vi "Async VI Control_Stop Processes.vi"(5 "Iterations":i32=39, 11 "VI Refs":refnum<vi>[](array[refnum])) -> ()   [LabVIEW 2021, in "CANOpen Addon Engine.lvlib"]
uses:
  CANOpen Addon Engine.lvlib
panel:
  out "error out":errorcluster
  out "States":T1(array[ring])
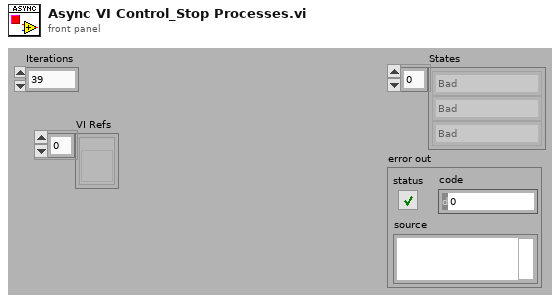
[diagram p1: front panel]
types:
  T1 = enum32{"Bad", "Idle", "Run top level", "Running"}[]
  T2 = enum32{"Bad", "Idle", "Run top level", "Running"}
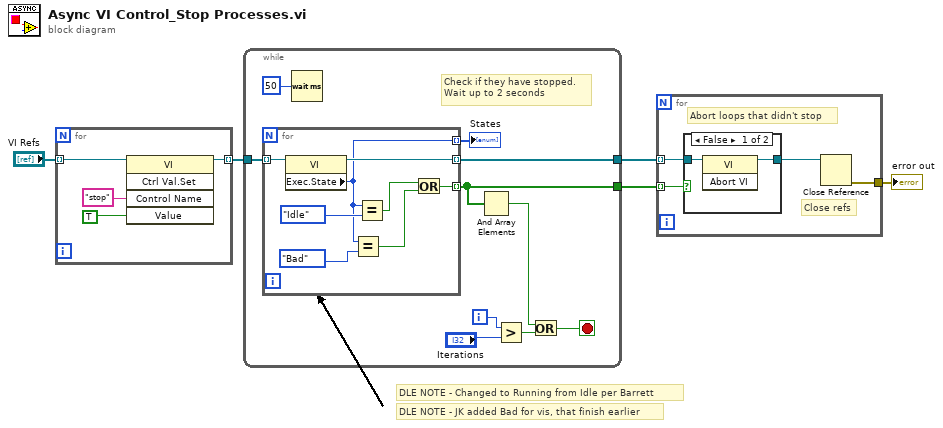
[diagram p0: block diagram]
diagram:
  # "DLE NOTE - JK added Bad for vis, that finish earlier"
  # "DLE NOTE - Changed to Running from Idle per Barrett"
  n1 = for {
    tunnel: "VI Refs" -> [w9] mode=indexing
    tunnel: [w7] -> w4 mode=indexing
    n2 = invoke class="VI" method="Ctrl Val.Set"(reference=w9, "Control Name"="stop", "Value"=TRUE ("force destroy? (F)")) -> (reference out=w7:refnum<vi>)  [unwired: 2 in, 4 out]
  }
  n3 = while {
    tunnel: w4 -> [w18]
    tunnel: [w17] -> w2
    tunnel: [w12] -> w3
    i -> [w15]
    stop <- w16 stop-if-true
    # "Check if they have stopped.\nWait up to 2 seconds"
    n4 = for {
      tunnel: w18 -> [w27] mode=indexing
      tunnel: [w22] -> w12 mode=indexing
      tunnel: [w26] -> w17 mode=indexing
      tunnel: [w24] -> w10 mode=indexing
      n5 = property class="VI"(reference=w27) -> (reference out=w26:refnum<vi>, "Exec.State"=w24:T2)  [unwired: 1 in, 1 out]
      n6 = Equal?(x=w24, y=T2."Bad") -> (x = y?=w20:bool)
      n7 = Equal?(x=w24, y=T2."Idle") -> (x = y?=w21:bool)
      n8 = Or(x=w21, y=w20) -> (x .or. y?=w22:bool)
    }
    "States" <- w10
    n9 = Wait (ms)(milliseconds to wait=u32 50) -> ()  [unwired: 1 out]
    n10 = And Array Elements(Boolean array=w12) -> (logical AND=w11:bool)
    n11 = Greater?(x=w15, y="Iterations") -> (0:w13:bool)
    n12 = Or(x=w11, y=w13) -> (x .or. y?=w16:bool)
  }
  n13 = for {
    tunnel: w2 -> [w31] mode=indexing
    tunnel: w3 -> [w30] mode=indexing
    tunnel: [w28] -> w1
    # "Close refs"
    # "Abort loops that didn't stop"
    n14 = case shown="False" w30 {
      tunnel: w31 -> [w33 w34]
      tunnel: [w32 w34] -> w29
      frame False {
        n15 = invoke class="VI" method="Abort VI"(reference=w33) -> (reference out=w32:refnum<vi>)  [unwired: 2 in, 2 out]
      }
      frame True {
      }
    }
    n16 = Close Reference(reference=w29) -> (error out=w28:errorcluster)  [unwired: 1 in]
  }
  "error out" <- w1
